vi "labview prueba tania 2.vi"() -> ()   [LabVIEW 2013]
panel:
  out "Contador":dbl
  out "Temperatura Mayor":dbl
  out "Temp Promedio":dbl
  out "Mucha calor":bool
  out "Thermometer":dbl(slide) scale=0.0..60.0
  # "Se tiene que generar la temperatura de todo un dia \nen intervalos de 2 horas, al final del dia debera de presentar\nla temperatura promedio de las temperaturas mayores a 35 grados \ny controlarlas.\nAl final del dia presentar la temperatura mayor.\nCuando la temperatura exceda los 40 grados debera de encender un led.\nEl programa puede detenerse si hay una temperatura arriba de los 55 grados."
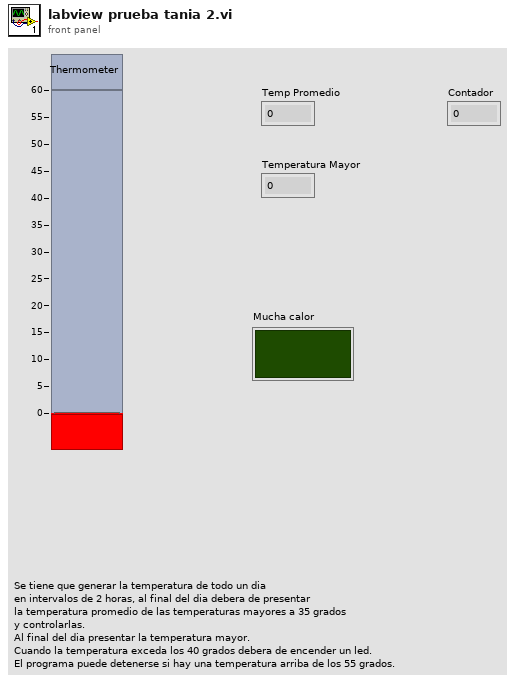
[diagram p1: front panel]
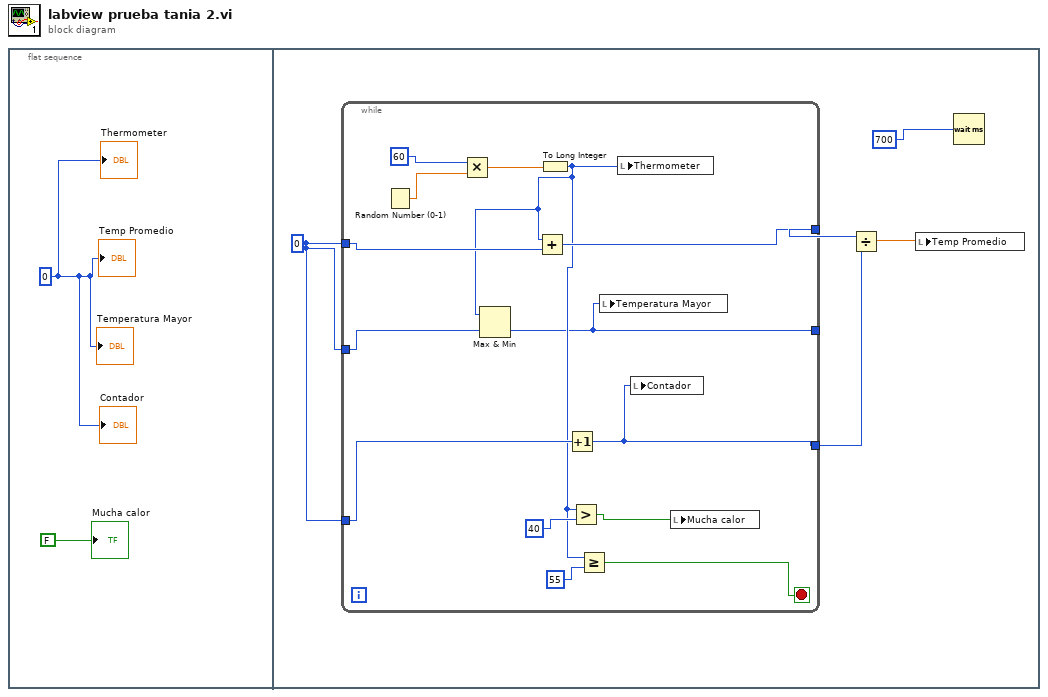
[diagram p0: block diagram]
diagram:
  n1 = flat-sequence {
    frame #0 {
      w2 = 0
      "Thermometer" <- w2
      "Temp Promedio" <- w2
      "Temperatura Mayor" <- w2
      "Contador" <- w2
      "Mucha calor" <- FALSE
    }
    frame #1 {
      w7 = 0
      n2 = while {
        tunnel: w7 -> [w18]
        tunnel: w7 -> [w16]
        tunnel: w7 -> [w15]
        tunnel: [w17] -> w6
        tunnel: [w14] -> w4
        tunnel: [w8] -> _
        stop <- w9 stop-if-true
        n3 = Random Number (0-1)() -> (number: 0 to 1=w20:dbl)
        n4 = Multiply(x=60, y=w20) -> (x*y=w19:dbl)
        n5 = To Long Integer(number=w19) -> (32bit integer=w11:i32)
        n6 = Max & Min(x=w11, y=w16) -> (min(x,y)=w8:i32)  [unwired: 1 out]
        n7 = Add(x=w11, y=w18) -> (x+y=w17:i32)
        n8 = Increment(x=w15) -> (x+1=w14:i32)
        n9 = Greater?(x=w11, y=40) -> (0:w12:bool)
        n10 = Greater Or Equal?(x=w11, y=55) -> (x >= y?=w9:bool)
        n11 = local write "Temperatura Mayor"(w8) -> ()
        n12 = local write "Thermometer"(w11) -> ()
        n13 = local write "Contador"(w14) -> ()
        n14 = local write "Mucha calor"(w12) -> ()
      }
      n15 = Divide(x=w6, y=w4) -> (x/y=w5:dbl)
      n16 = local write "Temp Promedio"(w5) -> ()
      n17 = Wait (ms)(milliseconds to wait=700) -> ()  [unwired: 1 out]
    }
  }
